vi "Create.vi"(8 "error in (no error)":errorcluster, 10 "ConfigurationFolder":path) -> (0 "error out":errorcluster, 3 "GCMConfigurationManager out":refnum<class "GCMConfigurationManager.lvclass">)   [LabVIEW 2014, in "GCMConfigurationManager.lvclass"]
uses:
  GCMConfigurationManager.lvclass
  GCMConfigurationManager.lvclass/GCMConfigurationManager.ctl
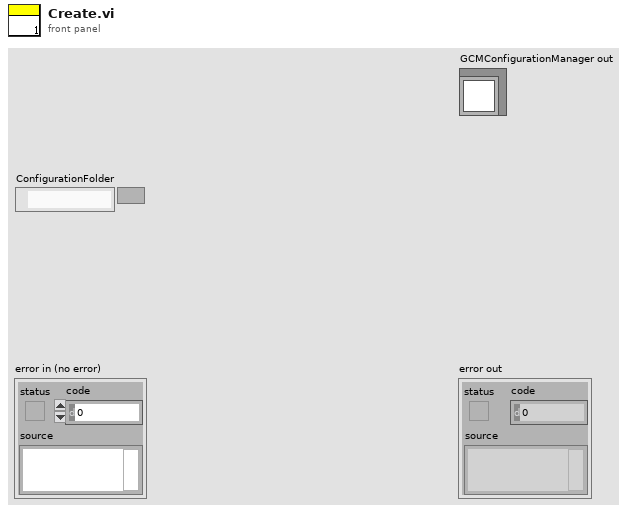
[diagram p1: front panel]
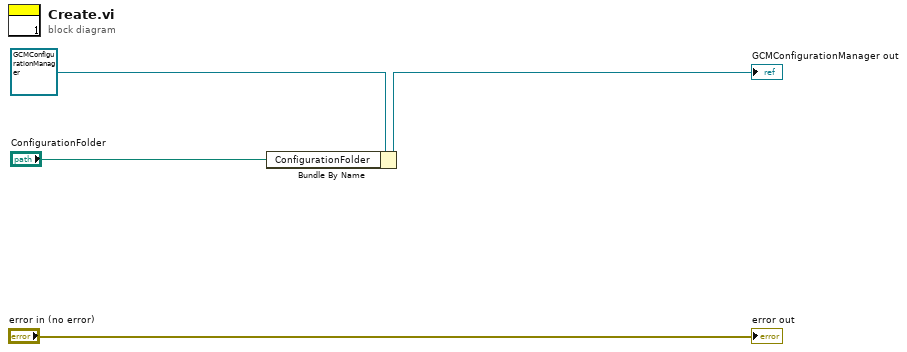
[diagram p0: block diagram]
diagram:
  n1 = Bundle By Name(cluster=refnum<class "GCMConfigurationManager.lvclass"> refnum ("GCMConfigurationManager in"), "ConfigurationFolder"="ConfigurationFolder") -> (→"GCMConfigurationManager out":refnum<class "GCMConfigurationManager.lvclass">)
  "error out" <- "error in (no error)"
